vi "D-Link Track Colour.vi"(10 "Image Dst":T1, 11 "New Image":T1) -> (1 "Object found?":bool, 2 "Object Output":cluster{"X":i32, "Y":i32}, 3 "Image Out":T1)   [LabVIEW 2012]
uses:
  <vilib>/vision/Image Controls.llb/IMAQ Image.ctl
  <vilib>/vision/NI_Vision_Development_Module.lvlib
panel:
  in  "Area Lower Limit":dbl=2000.0
  in  "Area Upper Limit":dbl=40000.0
  out "Blob Area":dbl
  in  "Show Image":bool
  out "Camera":T1(plugin-control)
  out "Particle Measurements (Pixels)":dbl[][](array[numeric]) format="%.2f"
  in  "Blue or Luma or Val or Inten Range":cluster{"Lower value":i32, "Upper value":i32}={"Lower value"=17, "Upper value"=200}
  in  "Green or Sat Range":cluster{"Lower value":i32, "Upper value":i32}={"Lower value"=17, "Upper value"=200}
  in  "Red or Hue Range":cluster{"Lower value":i32, "Upper value":i32}={"Lower value"=17, "Upper value"=200}
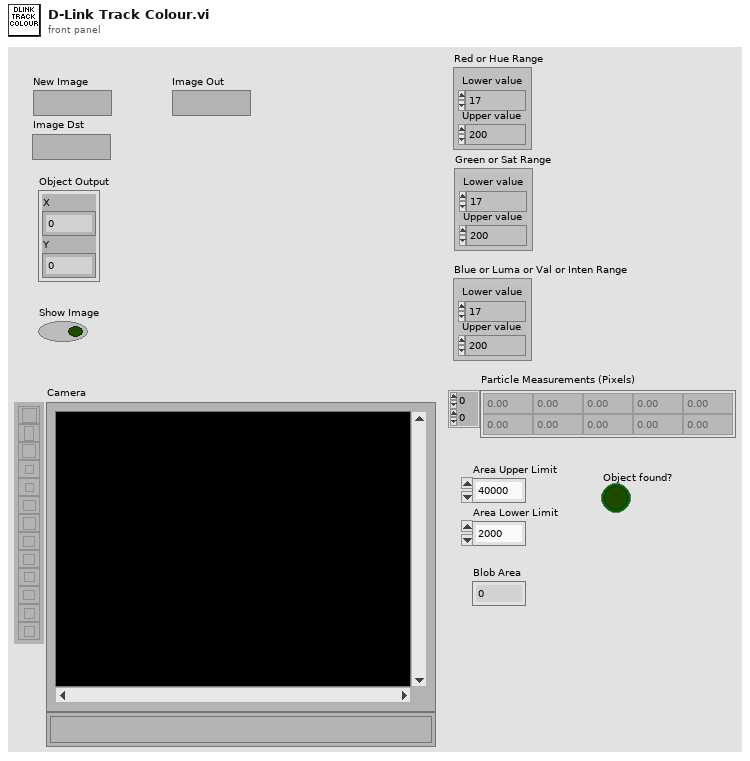
[diagram p1: front panel]
types:
  T1 = typedef "IMAQ Image.ctl" = refnum<image>
  T2 = cluster{"X Velocity (m/s)":dbl, "Y Velocity (m/s)":dbl, "Angular Velocity (rad/s)":dbl}
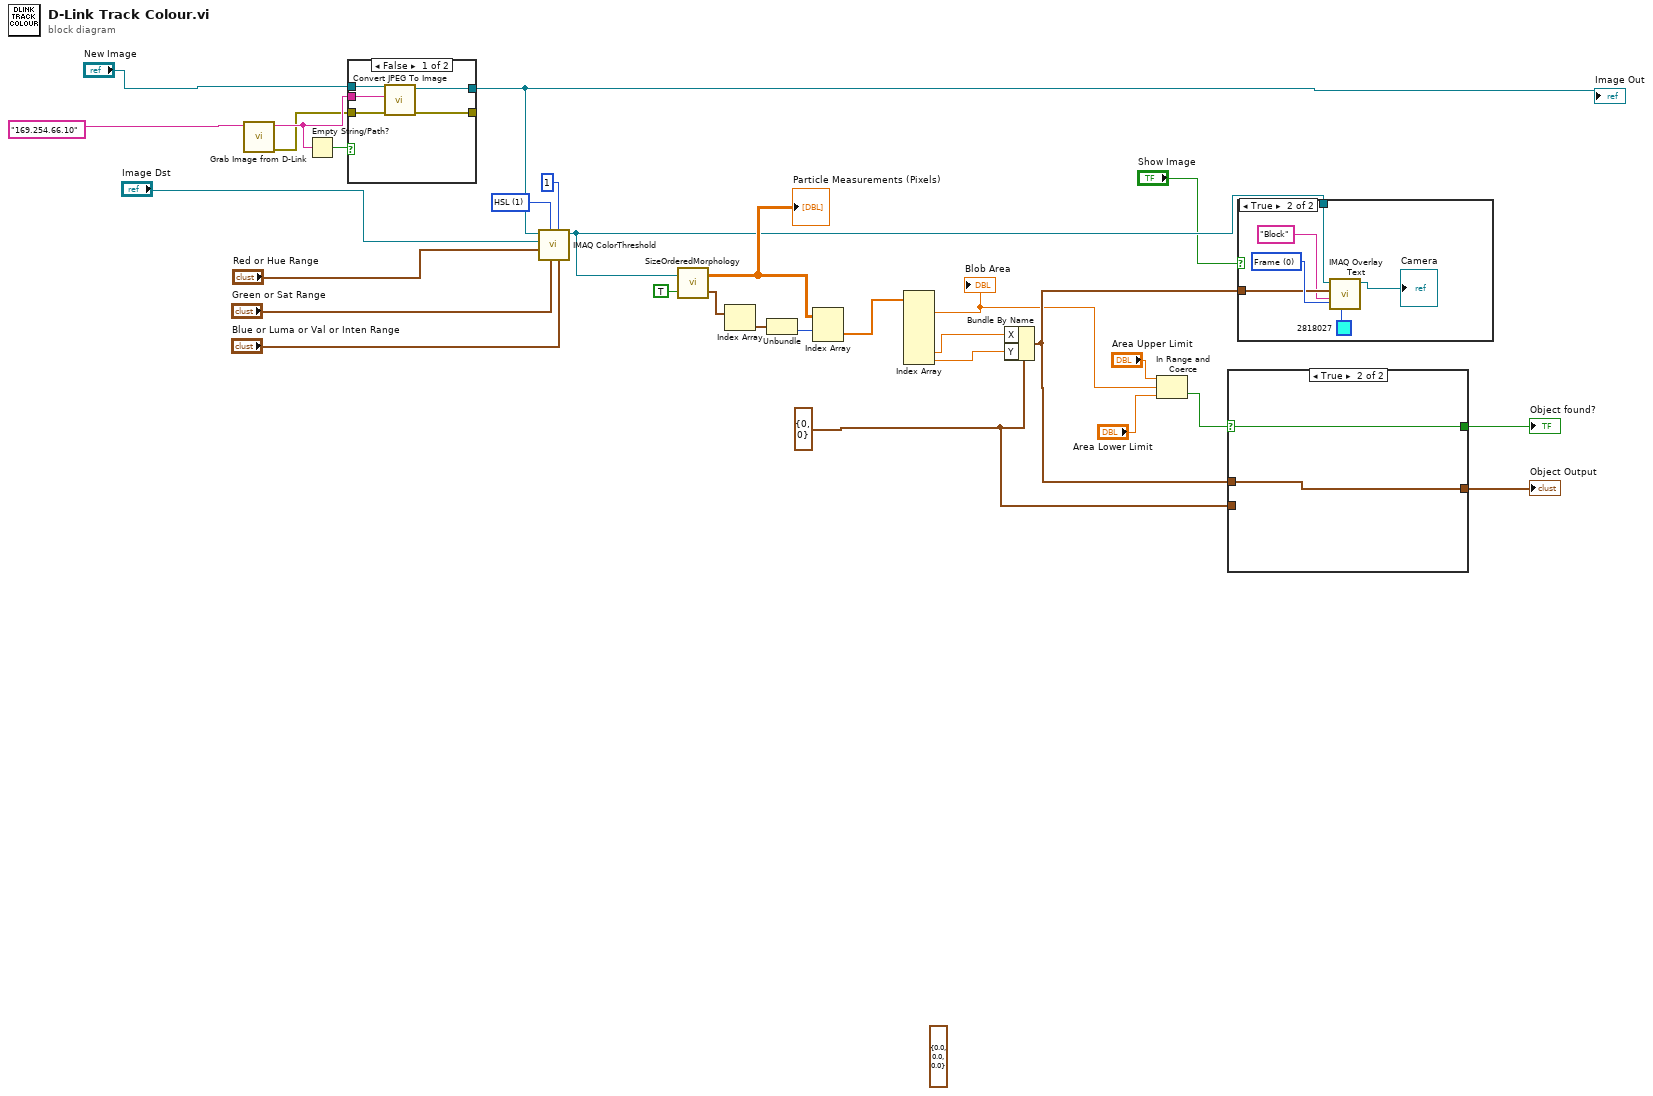
[diagram p0: block diagram]
diagram:
  w25 = u16 1 items=["RGB", "HSL", "HSV", "HSI"] ("Color Mode")
  (unwired) T2 {"X Velocity (m/s)"=0.0, "Y Velocity (m/s)"=0.0, "Angular Velocity (rad/s)"=0.0} ("Robot Velocities")
  w6 = cluster{"X":i32, "Y":i32} {"X"=0, "Y"=0} ("Origin")
  n1 = call "Grab Image from D-Link.vi"("address"="169.254.66.10") -> ("error out"=w27:errorcluster, "data out"=w28:string)  [unwired: 9 in]
  n2 = Empty String/Path?(string/path=w28) -> (empty?=w29:bool)
  n3 = case shown="False" w29 {
    tunnel: "New Image" -> [w35 w36]
    tunnel: w28 -> [w34 _]
    tunnel: w27 -> [w33 w37]
    tunnel: [w32 w37] -> _
    tunnel: [w31 w36] -> w30
    frame False {
      n4 = call "Convert JPEG To Image.vi"("error in"=w33, "Compressed Image"=w34, "Image In"=w35) -> ("error out"=w32:errorcluster, "Image Out"=w31:T1)  [unwired: 7 in]
    }
    frame True {
    }
  }
  "Image Out" <- w30
  n5 = call "IMAQ ColorThreshold"("Blue or Luma or Val or Inten Range"="Blue or Luma or Val or Inten Range", "Replace Value"=1, "Green or Sat Range"="Green or Sat Range", "Color Mode"=w25, "Red or Hue Range"="Red or Hue Range", "Image Dst"="Image Dst", "Image Src"=w30) -> ("Image Dst Out"=w12:T1)  [unwired: 3 in, 1 out]
  n6 = call "SizeOrderedMorphology.vi"("Green"=TRUE, "Image Dst Out"=w12) -> ("Sort Array"=w19:cluster{"Numeric":dbl, i32}[], "Particle Measurements (Pixels)"=w15:dbl[][])
  "Particle Measurements (Pixels)" <- w15
  n7 = Index Array(array=w19) -> (element=w18:cluster{"Numeric":dbl, i32})  [unwired: 1 in]
  n8 = Unbundle(w18) -> (w17:i32)  [unwired: 1 out]
  n9 = Index Array(array=w15, index (row)=w17) -> (element=w16:dbl[])  [unwired: 1 in]
  n10 = Index Array(array=w16) -> (element #1=w4:dbl, element #6=w13:dbl, element #7=w14:dbl)  [unwired: 7 in, 4 out]
  "Blob Area" <- w4
  n11 = Bundle By Name(cluster=w6, "X"=w13, "Y"=w14) -> (w22:cluster{"X":i32, "Y":i32})
  n12 = In Range and Coerce(upper limit="Area Upper Limit", x=w4, lower limit="Area Lower Limit") -> (In Range?=w5:bool)  [unwired: 1 out]
  n13 = case shown="True" w5 {
    selector: w5 -> [w38 w40]
    tunnel: w22 -> [_ w41]
    tunnel: [w39 w41] -> w7
    tunnel: w6 -> [w39 _]
    tunnel: [w38 w40] -> w1
    frame False {
    }
    frame True {
    }
  }
  "Object Output" <- w7
  "Object found?" <- w1
  n14 = case shown="True" "Show Image" {
    tunnel: w22 -> [_ w45]
    tunnel: w12 -> [_ w42]
    frame False {
    }
    frame True {
      w46 = u32 0 items=["Frame", "Fill", "Highlight"] ("Drawing Mode (Frame)")
      n15 = call "IMAQ Overlay Text"("BG Color (Transparent)"=w46, "Text Color (black)"=u32 2818027 ("Color"), "String"="Block", "Origin"=w45, "Image"=w42) -> ("Image Out"=→"Camera":T1)  [unwired: 5 in, 1 out]
    }
  }
